vi "example_3_5_b.vi"() -> ()   [LabVIEW 2018]
panel:
  out "Array":string[](array[string])
  # "NOTE: remember plug the Led Analyser\nbefore run LabVIEW and to change the\nVISA resource name in the schematic,\notherwise the application will not work."
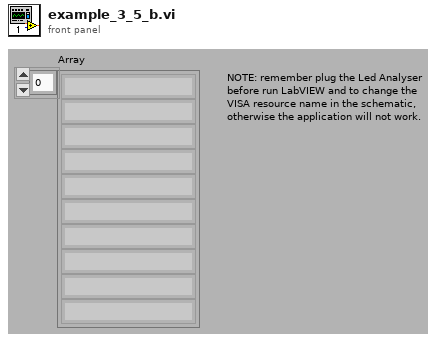
[diagram p1: front panel]
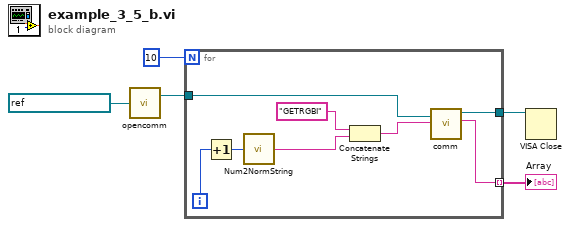
[diagram p0: block diagram]
diagram:
  n1 = call "opencomm.vi"("VISA resource name"=refnum<visa-resource-name> "ASRL20::INSTR") -> ("duplicate VISA resource name"=w4:refnum<visa-resource-name>)  [unwired: 1 out]
  n2 = for {
    N: 10 -> [_]
    tunnel: w4 -> [w13]
    tunnel: [w12] -> w3
    tunnel: [w11] -> w1 mode=indexing
    i -> [w6]
    n3 = Increment(x=w6) -> (x+1=w7:i32)
    n4 = call "Num2NormString.vi"("Number"=w7) -> ("Normalized String Number"=w8:string)
    n5 = Concatenate Strings("GETRGBI" ("Command"), w8) -> (w9:string)
    n6 = call "comm.vi"("VISA resource name"=w13, "Command"=w9) -> ("dup VISA resource name"=w12:refnum<visa-resource-name>, "Response"=w11:string)  [unwired: 2 out]
  }
  "Array" <- w1
  n7 = VISA Close(VISA resource name=w3) -> ()  [unwired: 1 in, 1 out]
